vi "CoincidenceBuildImage.vi"(11 "notes 2":refnum<vi>) -> ()   [LabVIEW 2009]
uses:
  <vilib>/Analysis/NI_AALPro.lvlib
panel:
  out "Waveform Graph":i32[](graph)
  out "Array":i32[](array[numeric])
  in  "square":bool
  in  "ratio":bool caption="Nc"
  in  "y":i32(listbox)
  in  "notes":string
  out "Ampel":cluster{"RED":bool, "YELLOW":bool, "GREEN":bool}
  in  "threshold":u32=30
  in  "Color Palette":T1(ring)
  in  "START":bool
  in  "stop":bool
  in  "new Pixelsize\nx":i32(listbox)
  in  "coincidence settings":T2={"length [µs]"=10.0, "delayed channel"=0, "center peak (µs)"=0.6, "lateral peaks"=2} {"lateral peaks" min=2 max=10 step=2; "center peak (µs)" format="%.2f"; "length [µs]" format="%.2f"}
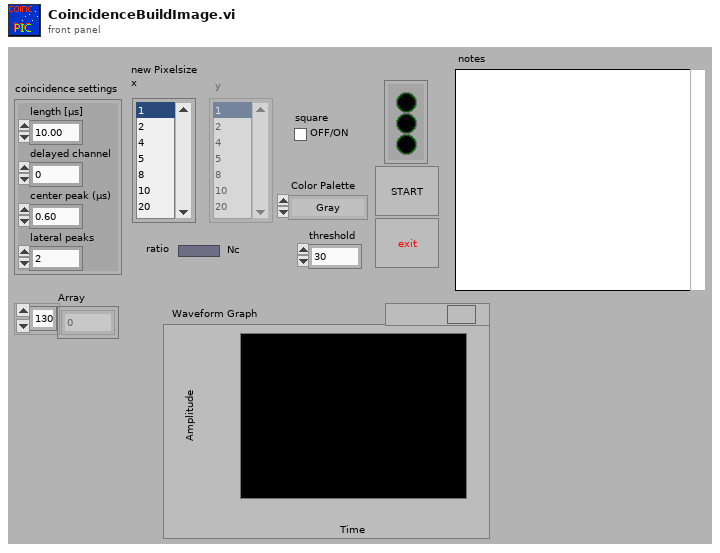
[diagram p1: front panel]
types:
  T1 = enum32{"Gray", "Binary", "Gradient", "Rainbow", "Temperature"}
  T2 = cluster{"length [µs]":dbl, "delayed channel":u8, "center peak (µs)":dbl, "lateral peaks":u32}
  T3 = typedef "ImageSettings.ctt" = cluster{"Start Position (µm)":cluster{"x":dbl, "y":dbl, "z":dbl}, "End Position (µm)":cluster{"x":dbl, "y":dbl, "z":dbl}, "Image Resolution (nm/pixel)":cluster{"x":dbl, "y":dbl, "z":dbl}, "Image Size (µm)":cluster{"x":dbl, "y":dbl, "z":dbl}, "Image Size (pixel)":cluster{"x":u32, "y":u32, "z":u32}, "Time Resolution\n(ms/pixel)":dbl, "1st Axis":u16, "2nd Axis":u16, "Retrace":bool, "Estimated Time":string}
  T4 = enum16{"Ini", "Get", "Set", "Draw", "Colorpal", "Dump", "Zoom"}
  T5 = cluster{"new image dim":i32, "new image dim":i32}
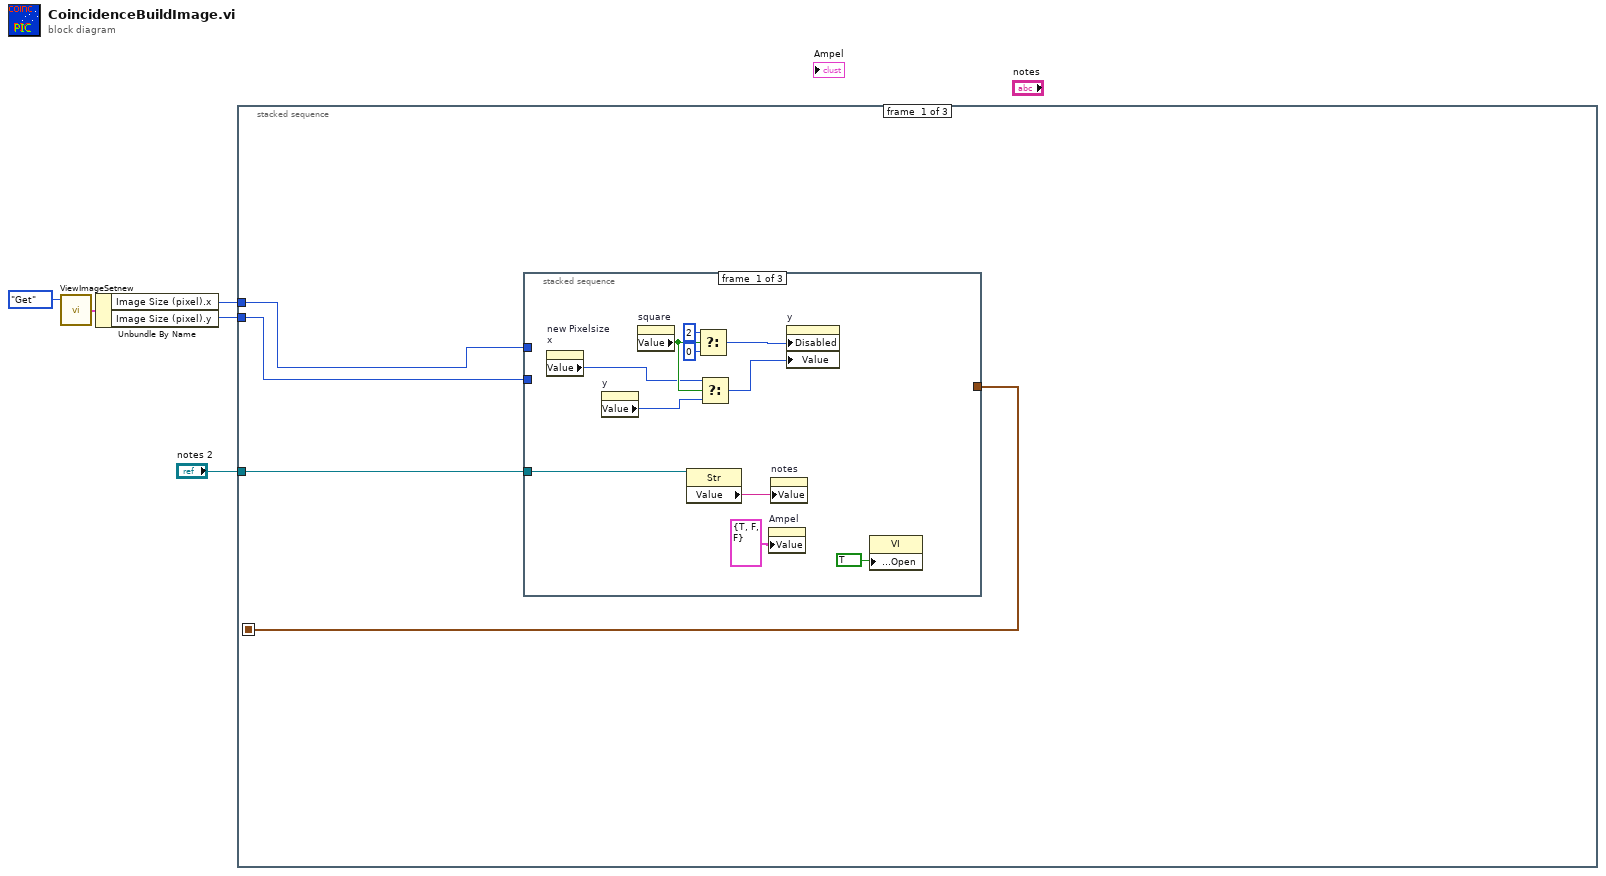
[diagram p0: block diagram]
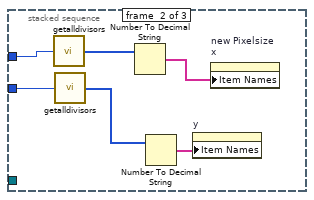
[diagram p2: hidden frame]
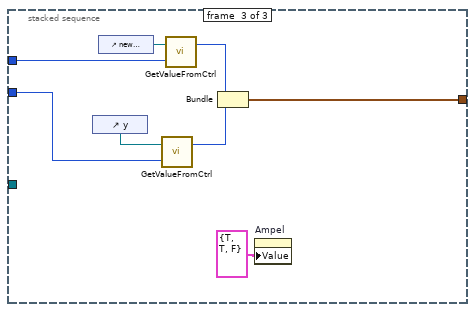
[diagram p3: hidden frame]
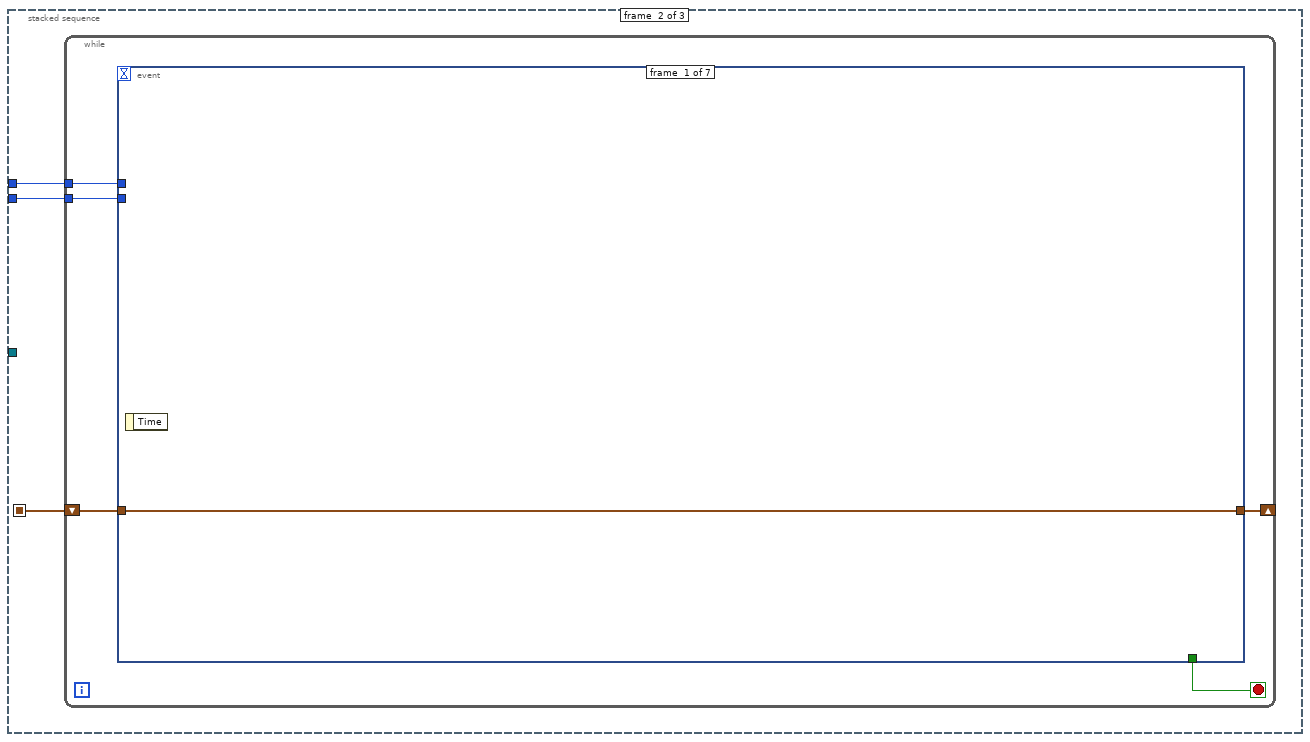
[diagram p4: hidden frame]
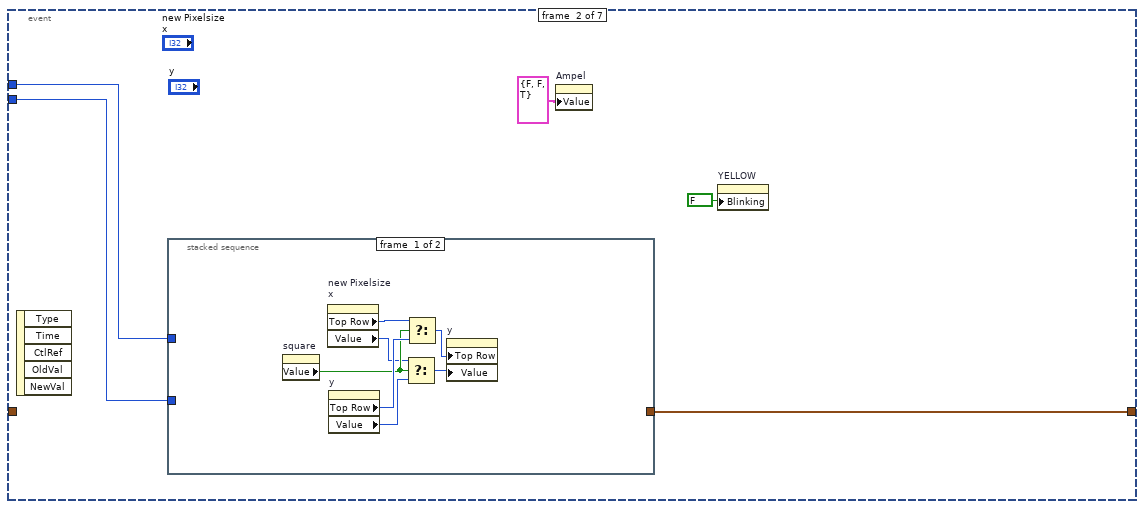
[diagram p5: hidden frame]
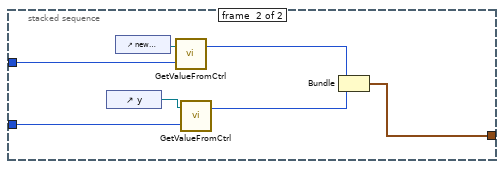
[diagram p6: hidden frame]
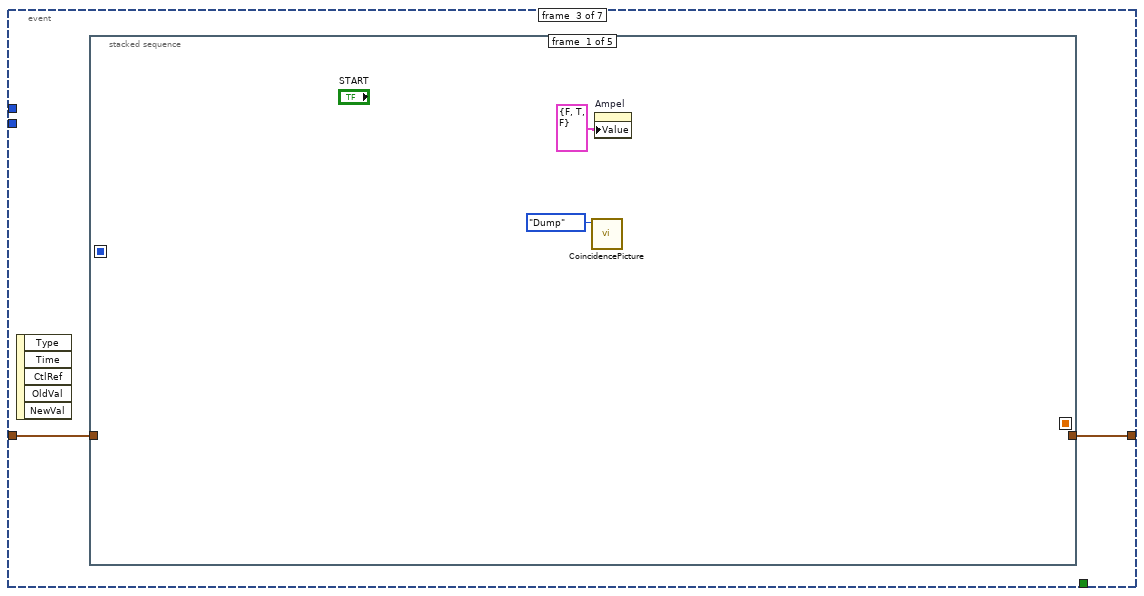
[diagram p7: hidden frame]
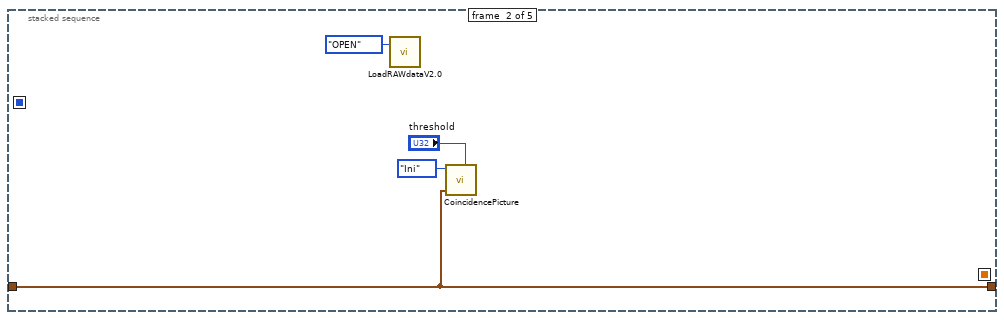
[diagram p8: hidden frame]
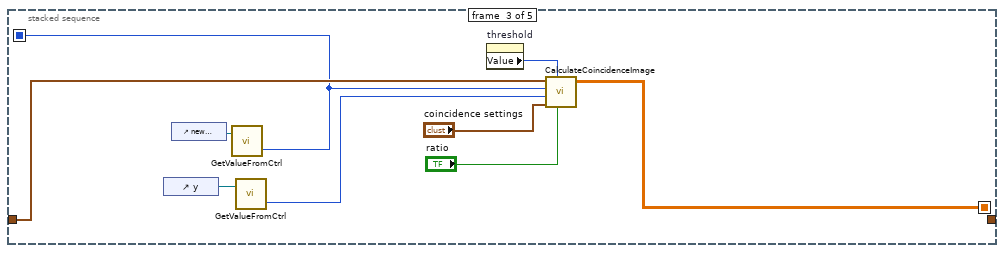
[diagram p9: hidden frame]
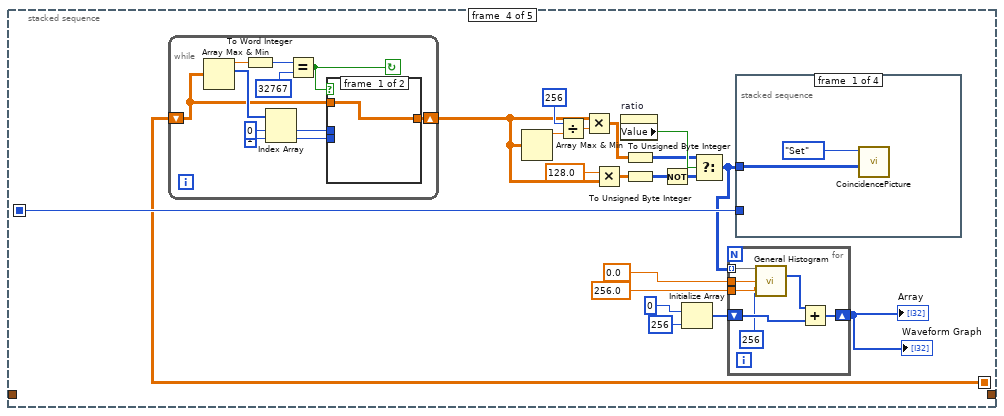
[diagram p10: hidden frame]
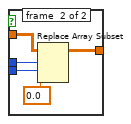
[diagram p11: hidden frame]
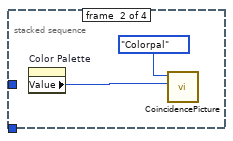
[diagram p12: hidden frame]
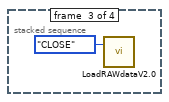
[diagram p13: hidden frame]
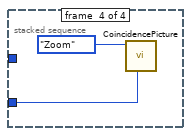
[diagram p14: hidden frame]
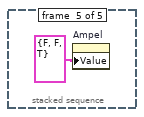
[diagram p15: hidden frame]
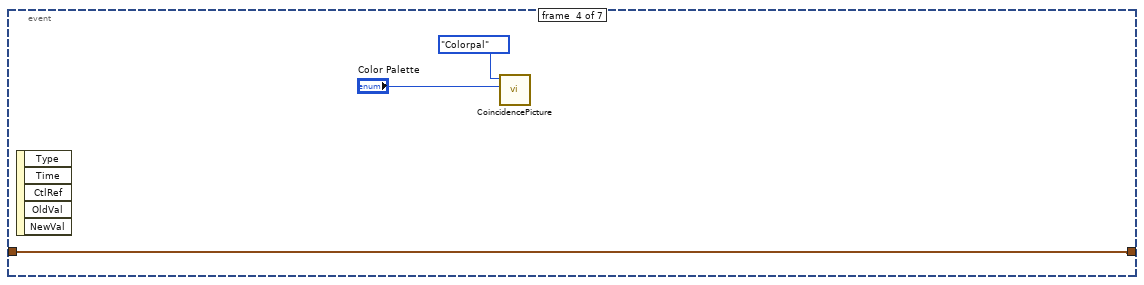
[diagram p16: hidden frame]
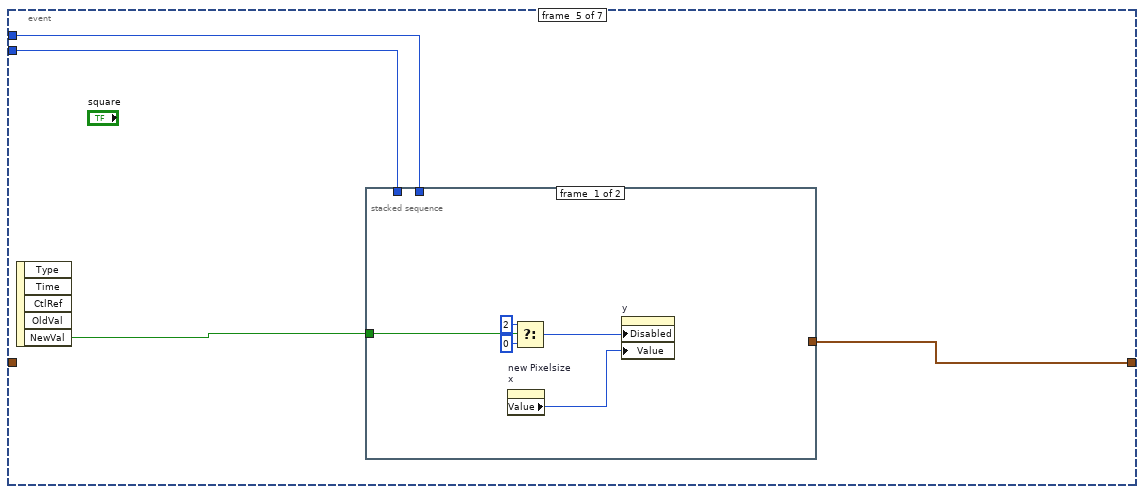
[diagram p17: hidden frame]
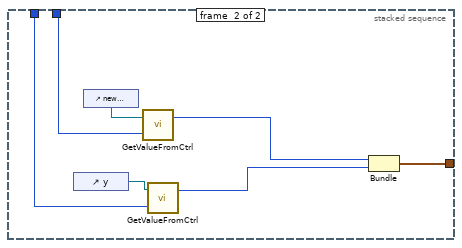
[diagram p18: hidden frame]
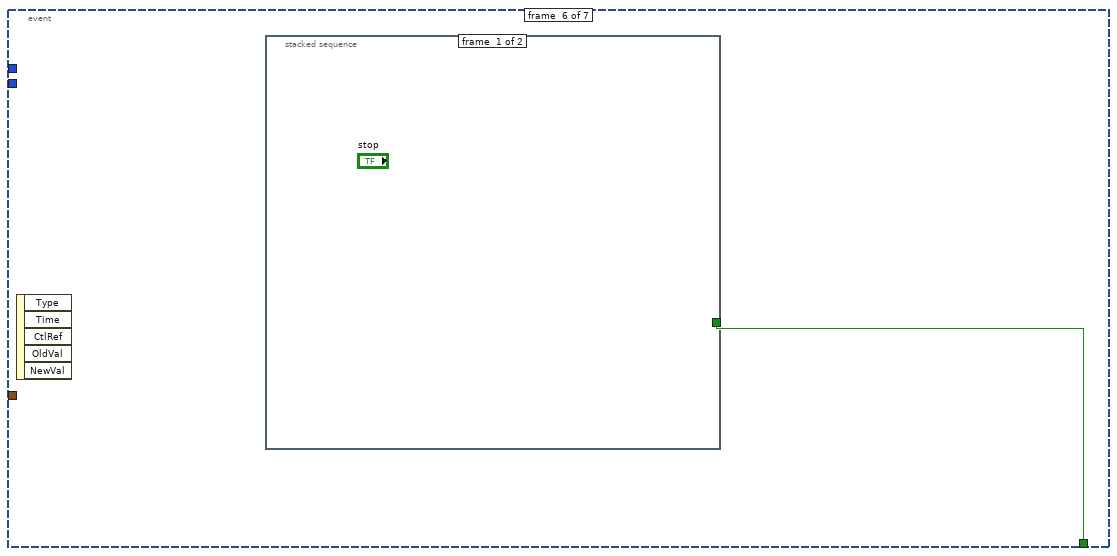
[diagram p19: hidden frame]
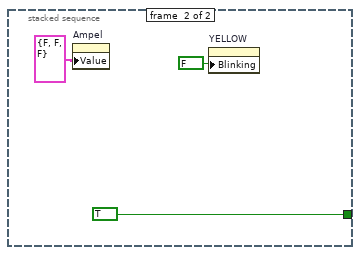
[diagram p20: hidden frame]
diagram:
  n1 = call "ViewImageSetnew.vi"("action"=enum16{"Display", "change", "Get", "Set"}."Get" ("Enum")) -> ("Image Settings"=w2:T3)  [unwired: 2 in]
  n2 = Unbundle By Name(w2) -> ("Image Size (pixel).x"=w1:u32, "Image Size (pixel).y"=w4:u32)
  n3 = stacked-sequence {
    seq-local: [w6 _ _] -> [_ w35 _]
    tunnel: "notes 2" -> [w9 _ w156]
    tunnel: w1 -> [w8 w37 _]
    tunnel: w4 -> [w7 w36 _]
    frame #0 {
      n4 = stacked-sequence {
        tunnel: w8 -> [_ w26 w31]
        tunnel: w7 -> [_ w25 w32]
        tunnel: w9 -> [w17 _ _]
        tunnel: [_ _ w27] -> w6
        frame #0 {
          n5 = property on="new Pixelsize\nx" class="LstBox (strict)"() -> ("Value"=w11:i32)  [unwired: 2 in, 2 out]
          n6 = property on="y" class="LstBox (strict)"() -> ("Value"=w12:i32)  [unwired: 2 in, 2 out]
          n7 = property on="square" class="Boolean (strict)"() -> ("Value"=w13:bool)  [unwired: 2 in, 2 out]
          n8 = property class="Str"(reference=w17) -> ("Value"=w18:string)  [unwired: 1 in, 2 out]
          n9 = Select(t=u8 2 ("Disabled"), s=w13, f=u8 0 ("Disabled")) -> (s? t:f=w16:u8)
          n10 = Select(t=w11, s=w13, f=w12) -> (s? t:f=w10:i32)
          n11 = property on="Ampel" class="Cluster (strict)"("Value"=cluster{"RED":bool, "YELLOW":bool, "GREEN":bool} {"RED"=TRUE, "YELLOW"=FALSE, "GREEN"=FALSE} ("Ampel")) -> ()  [unwired: 2 in, 2 out]
          n12 = property on="notes" class="String"("Value"=w18) -> ()  [unwired: 2 in, 2 out]
          n13 = property on="y" class="LstBox (strict)"("Disabled"=w16, "Value"=w10) -> ()  [unwired: 2 in, 2 out]
          n14 = property class="VI"("Front Panel Window:Open"=TRUE) -> ()  [unwired: 2 in, 2 out]
        }
        frame #1 {
          n15 = call "getalldivisors.vi"("x"=w26) -> ("Array"=w23:i32[])
          n16 = call "getalldivisors.vi"("x"=w25) -> ("Array"=w24:i32[])
          n17 = Number To Decimal String(number=w23) -> (decimal integer string=w21:string[])  [unwired: 1 in]
          n18 = Number To Decimal String(number=w24) -> (decimal integer string=w22:string[])  [unwired: 1 in]
          n19 = property on="y" class="LstBox (strict)"("Item Names"=w22) -> ()  [unwired: 2 in, 2 out]
          n20 = property on="new Pixelsize\nx" class="LstBox (strict)"("Item Names"=w21) -> ()  [unwired: 2 in, 2 out]
        }
        frame #2 {
          n21 = control-ref of="y"() -> (w33:refnum<vi>)
          n22 = control-ref of="new Pixelsize\nx"() -> (w30:refnum<vi>)
          n23 = call "GetValueFromCtrl.vi"("imagesize"=w32, "new pixelsize ctrl"=w33) -> ("new image dim"=w28:i32)  [unwired: 1 out]
          n24 = call "GetValueFromCtrl.vi"("imagesize"=w31, "new pixelsize ctrl"=w30) -> ("new image dim"=w29:i32)  [unwired: 1 out]
          n25 = Bundle("new image dim"=w29, "new image dim"=w28) -> (w27:T5)  [unwired: 1 in]
          n26 = property on="Ampel" class="Cluster (strict)"("Value"=cluster{"RED":bool, "YELLOW":bool, "GREEN":bool} {"RED"=TRUE, "YELLOW"=TRUE, "GREEN"=FALSE} ("Ampel")) -> ()  [unwired: 2 in, 2 out]
        }
      }
    }
    frame #1 {
      n27 = while {
        shift-right: [w41] -> _
        shift-left: w35 -> [w40]
        tunnel: w37 -> [w39]
        tunnel: w36 -> [w38]
        stop <- w42 stop-if-true
        n28 = event shown="[2] \"START\": Value Change" {
          selector: _ -> [_ _ _ _ _ _ _]
          dyn-events: _ -> [_ _ _ _ _ _ _]
          timeout: _ -> [_ _ _ _ _ _ _]
          tunnel: [_ _ _ _ _ w151 TRUE] -> w42
          tunnel: [w43 w44 w63 w132 w137 _ _] -> w41
          tunnel: w40 -> [w43 _ w64 w132 _ _ _]
          tunnel: w39 -> [_ w45 _ _ w135 _ _]
          tunnel: w38 -> [_ w46 _ _ w138 _ _]
          event #0 {
            n29 = event-data() -> ()  [unwired: 1 in, 1 out]
          }
          event #1 {
            n30 = event-data() -> ()  [unwired: 1 in, 5 out]
            n31 = stacked-sequence {
              tunnel: w46 -> [_ w56]
              tunnel: w45 -> [_ w57]
              tunnel: [_ w62] -> w44
              frame #0 {
                n32 = property on="square" class="Boolean (strict)"() -> ("Value"=w51:bool)  [unwired: 2 in, 2 out]
                n33 = property on="new Pixelsize\nx" class="LstBox (strict)"() -> ("Top Row"=w52:i32, "Value"=w50:i32)  [unwired: 2 in, 2 out]
                n34 = property on="y" class="ListBox (strict)"() -> ("Top Row"=w55:i32, "Value"=w54:i32)  [unwired: 2 in, 2 out]
                n35 = Select(t=w50, s=w51, f=w54) -> (s? t:f=w49:i32)
                n36 = Select(t=w52, s=w51, f=w55) -> (s? t:f=w53:i32)
                n37 = property on="y" class="ListBox (strict)"("Top Row"=w53, "Value"=w49) -> ()  [unwired: 2 in, 2 out]
              }
              frame #1 {
                n38 = control-ref of="y"() -> (w60:refnum<vi>)
                n39 = control-ref of="new Pixelsize\nx"() -> (w61:refnum<vi>)
                n40 = call "GetValueFromCtrl.vi"("imagesize"=w57, "new pixelsize ctrl"=w61) -> ("new image dim"=w59:i32)  [unwired: 1 out]
                n41 = call "GetValueFromCtrl.vi"("imagesize"=w56, "new pixelsize ctrl"=w60) -> ("new image dim"=w58:i32)  [unwired: 1 out]
                n42 = Bundle("new image dim"=w59, "new image dim"=w58) -> (w62:T5)  [unwired: 1 in]
              }
            }
            n43 = property on="Ampel" class="Cluster (strict)"("Value"=cluster{"RED":bool, "YELLOW":bool, "GREEN":bool} {"RED"=FALSE, "YELLOW"=FALSE, "GREEN"=TRUE} ("Ampel")) -> ()  [unwired: 2 in, 2 out]
            n44 = property on="YELLOW" class="Boolean (strict)"("Blinking"=FALSE) -> ()  [unwired: 2 in, 2 out]
          }
          event #2 {
            n45 = event-data() -> ()  [unwired: 1 in, 5 out]
            n46 = stacked-sequence {
              seq-local: [_ _ w78 _ _] -> [_ _ _ w97 _]
              seq-local: [_ _ w73 _ _] -> [_ _ _ w98 _]
              tunnel: w64 -> [_ w70 w79 _ _]
              tunnel: [_ w70 _ _ _] -> w63
              frame #0 {
                n47 = call "CoincidencePicture.vi"("Enum"=T4."Dump") -> ()  [unwired: 6 in, 3 out]
                n48 = property on="Ampel" class="Cluster (strict)"("Value"=cluster{"RED":bool, "YELLOW":bool, "GREEN":bool} {"RED"=FALSE, "YELLOW"=TRUE, "GREEN"=FALSE} ("Ampel")) -> ()  [unwired: 2 in, 2 out]
              }
              frame #1 {
                n49 = call "LoadRAWdataV2.0.vi"("action"=enum16{"OPEN", "READ", "CLOSE"}."OPEN" ("Enum")) -> ()  [unwired: 1 in, 2 out]
                n50 = call "CoincidencePicture.vi"("threshold"="threshold", "new IMAGElsize"=w70, "Enum"=T4."Ini") -> ()  [unwired: 4 in, 3 out]
              }
              frame #2 {
                n51 = control-ref of="y"() -> (w72:refnum<vi>)
                n52 = control-ref of="new Pixelsize\nx"() -> (w74:refnum<vi>)
                n53 = call "GetValueFromCtrl.vi"("new pixelsize ctrl"=w74) -> ("value"=w73:i32)  [unwired: 1 in, 1 out]
                n54 = call "GetValueFromCtrl.vi"("new pixelsize ctrl"=w72) -> ("value"=w71:i32)  [unwired: 1 in, 1 out]
                n55 = property on="threshold" class="DigNum (strict)"() -> ("Value"=w77:u32)  [unwired: 2 in, 2 out]
                n56 = call "CalculateCoincidenceImage.vi"("new dimension"=w79, "threshold"=w77, "new pixelsize x"=w73, "newpixelsize y"=w71, "ratio"="ratio", "coincidence settings"="coincidence settings") -> ("result"=w78:dbl[][])  [unwired: 2 in]
              }
              frame #3 {
                n57 = while {
                  shift-right: [w107] -> w83
                  shift-left: w97 -> [w108]
                  stop <- w114 continue-if-true
                  n58 = Array Max & Min(array=w108) -> (max value=w117:dbl, max index (indices)=w113:i32[])  [unwired: 2 out]
                  n59 = To Word Integer(number=w117) -> (16bit integer=w115:i16)
                  n60 = Index Array(array=w113, index #1=0 ("index"), index #2=1 ("index")) -> (element #1=w110:i32, element #2=w109:i32)
                  n61 = Equal?(x=w115, y=i16 32767) -> (x = y?=w114:bool)
                  n62 = case shown="True" w114 {
                    tunnel: w108 -> [w118 w123]
                    tunnel: w110 -> [_ w122]
                    tunnel: w109 -> [_ w121]
                    tunnel: [w118 w119] -> w107
                    frame #0 {
                    }
                    frame #1 {
                      n63 = Replace Array Subset(array=w123, new element=0.0 ("new element/subarray"), index (row)=w122, index (col)=w121) -> (w119:dbl[][])
                    }
                  }
                }
                n64 = Array Max & Min(array=w83) -> (max value=w88:dbl)  [unwired: 3 out]
                n65 = Divide(x=256, y=w88) -> (x/y=w91:dbl)
                n66 = Multiply(x=w83, y=w91) -> (x*y=w90:dbl[][])
                n67 = Multiply(x=128.0 ("y"), y=w83) -> (x*y=w99:dbl[][])
                n68 = property on="ratio" class="Bool (strict)"() -> ("Value"=w95:bool)  [unwired: 2 in, 2 out]
                n69 = To Unsigned Byte Integer(number=w90) -> (unsigned 8bit integer=w92:u8[][])
                n70 = To Unsigned Byte Integer(number=w99) -> (unsigned 8bit integer=w93:u8[][])
                n71 = Not(x=w93) -> (.not. x?=w94:u8[][])
                n72 = Initialize Array(0, 256 ("dimension size")) -> (w86:i32[])
                n73 = Select(t=w92, s=w95, f=w94) -> (s? t:f=w82:u8[][])
                n74 = for {
                  tunnel: w82 -> [w106] mode=indexing
                  shift-right: [w105] -> w87
                  shift-left: w86 -> [w103]
                  tunnel: 0.0 ("max") -> [w101]
                  tunnel: 256.0 ("max") -> [w100]
                  n75 = call <vilib>:"General Histogram.vi"("X"=w106, "max"=w101, "min"=w100, "# bins"=256) -> ("Histogram"=w104:i32[])  [unwired: 7 in, 4 out]
                  n76 = Add(x=w104, y=w103) -> (x+y=w105:i32[])
                }
                "Array" <- w87
                "Waveform Graph" <- w87
                n77 = stacked-sequence {
                  tunnel: w82 -> [w124 _ _ _]
                  tunnel: w98 -> [_ _ _ w129]
                  frame #0 {
                    n78 = call "CoincidencePicture.vi"("Image Pixels (U8)"=w124, "Enum"=T4."Set") -> ()  [unwired: 5 in, 3 out]
                  }
                  frame #1 {
                    n79 = property on="Color Palette" class="Enum (strict)"() -> ("Value"=w127:T1)  [unwired: 2 in, 2 out]
                    n80 = call "CoincidencePicture.vi"("Palette Number (gray)"=w127, "Enum"=T4."Colorpal") -> ()  [unwired: 5 in, 3 out]
                  }
                  frame #2 {
                    n81 = call "LoadRAWdataV2.0.vi"("action"=enum16{"OPEN", "READ", "CLOSE"}."CLOSE" ("Enum")) -> ()  [unwired: 1 in, 2 out]
                  }
                  frame #3 {
                    n82 = call "CoincidencePicture.vi"("Zoom"=w129, "Enum"=T4."Zoom") -> ()  [unwired: 5 in, 3 out]
                  }
                }
              }
              frame #4 {
                n83 = property on="Ampel" class="Cluster (strict)"("Value"=cluster{"RED":bool, "YELLOW":bool, "GREEN":bool} {"RED"=FALSE, "YELLOW"=FALSE, "GREEN"=TRUE} ("Ampel")) -> ()  [unwired: 2 in, 2 out]
              }
            }
          }
          event #3 {
            n84 = event-data() -> ()  [unwired: 1 in, 5 out]
            n85 = call "CoincidencePicture.vi"("Palette Number (gray)"="Color Palette", "Enum"=enum16{"Ini", "Get", "Set", "Draw", "Colorpal"}."Colorpal") -> ()  [unwired: 5 in, 3 out]
          }
          event #4 {
            n86 = event-data() -> ("NewVal"=w136:bool)  [unwired: 1 in, 4 out]
            n87 = stacked-sequence {
              tunnel: w138 -> [_ w147]
              tunnel: [_ w150] -> w137
              tunnel: w136 -> [w139 _]
              tunnel: w135 -> [_ w149]
              frame #0 {
                n88 = property on="new Pixelsize\nx" class="LstBox (strict)"() -> ("Value"=w143:i32)  [unwired: 2 in, 2 out]
                n89 = Select(t=u8 2 ("Disabled"), s=w139, f=u8 0 ("Disabled")) -> (s? t:f=w140:u8)
                n90 = property on="y" class="LstBox (strict)"("Disabled"=w140, "Value"=w143) -> ()  [unwired: 2 in, 2 out]
              }
              frame #1 {
                n91 = control-ref of="y"() -> (w146:refnum<vi>)
                n92 = control-ref of="new Pixelsize\nx"() -> (w148:refnum<vi>)
                n93 = call "GetValueFromCtrl.vi"("imagesize"=w149, "new pixelsize ctrl"=w148) -> ("new image dim"=w144:i32)  [unwired: 1 out]
                n94 = call "GetValueFromCtrl.vi"("imagesize"=w147, "new pixelsize ctrl"=w146) -> ("new image dim"=w145:i32)  [unwired: 1 out]
                n95 = Bundle("new image dim"=w144, "new image dim"=w145) -> (w150:T5)  [unwired: 1 in]
              }
            }
          }
          event #5 {
            n96 = event-data() -> ()  [unwired: 1 in, 5 out]
            n97 = stacked-sequence {
              tunnel: [_ TRUE] -> w151
              frame #0 {
              }
              frame #1 {
                n98 = property on="Ampel" class="Cluster (strict)"("Value"=cluster{"RED":bool, "YELLOW":bool, "GREEN":bool} {"RED"=FALSE, "YELLOW"=FALSE, "GREEN"=FALSE} ("Ampel")) -> ()  [unwired: 2 in, 2 out]
                n99 = property on="YELLOW" class="Boolean (strict)"("Blinking"=FALSE) -> ()  [unwired: 2 in, 2 out]
              }
            }
          }
          event #6 {
            n100 = event-data() -> ()  [unwired: 1 in, 3 out]
            n101 = event-data() -> ()  [unwired: 2 in, 1 out]
          }
        }
      }
    }
    frame #2 {
      n102 = property on="notes" class="String"() -> ("Value"=w157:string)  [unwired: 2 in, 2 out]
      n103 = property class="Str"(reference=w156, "Value"=w157) -> ()  [unwired: 1 in, 2 out]
      n104 = property class="VI"("Front Panel Window:Open"=FALSE) -> ()  [unwired: 2 in, 2 out]
    }
  }
